vi "RecordDataToEventProgressCounterUp.vi"(10 "RecordData":string[][](array[string]), 11 "EventProgressDataInput":string[][](array[string])) -> (3 "EventProgressDataOutput":string[][](array[string]))   [LabVIEW 2017]
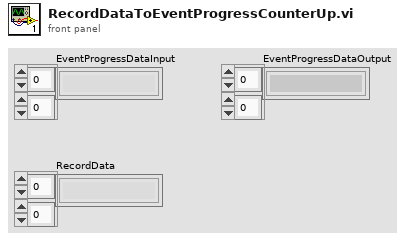
[diagram p1: front panel]
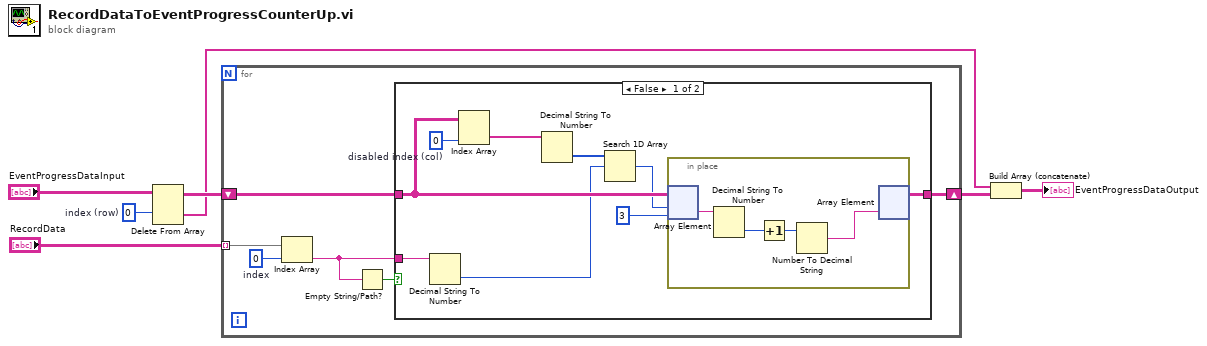
[diagram p0: block diagram]
diagram:
  w3 = 0  # index (row)
  n1 = Delete From Array "Delete From Array"(array="EventProgressDataInput", index (row)=w3) -> (deleted portion=w1:string[], array with subset deleted=w5:string[][])  [unwired: 2 in]
  n2 = for {
    tunnel: "RecordData" -> [w13] mode=indexing
    shift-right: [w10] -> w6
    shift-left: w5 -> [w12]
    w11 = 0  # index
    n3 = Index Array "Index Array"(array=w13, index=w11) -> (element=w9:string)
    n4 = Empty String/Path?(string/path=w9) -> (empty?=w8:bool)
    n5 = case shown="False" w8 {
      tunnel: w12 -> [w21 w27]
      tunnel: [w17 w27] -> w10
      tunnel: w9 -> [w14 _]
      frame False {
        w22 = 0  # disabled index (col)
        n6 = Decimal String To Number(string=w14) -> (number=w18:i32)  [unwired: 2 in, 1 out]
        n7 = Index Array "Index Array"(array=w21, index (col)=w22) -> (element=w20:string[])  [unwired: 1 in]
        n8 = Decimal String To Number(string=w20) -> (number=w19:i32[])  [unwired: 2 in, 1 out]
        n9 = Search 1D Array(1D array=w19, element=w18) -> (index of element=w16:i32)  [unwired: 1 in]
        n10 = in-place {
          n11 = in-place-array #1(w21, w16, 3) -> (w26:string)
          n12 = Decimal String To Number(string=w26) -> (number=w25:i32)  [unwired: 2 in, 1 out]
          n13 = Increment(x=w25) -> (x+1=w23:i32)
          n14 = Number To Decimal String(number=w23) -> (decimal integer string=w24:string)  [unwired: 1 in]
          n15 = in-place-array #1(w24) -> (w17:string[][])  [unwired: 2 out]
        }
      }
      frame True {
      }
    }
  }
  n16 = Build Array (concatenate) "Build Array"(w1, w6) -> (→"EventProgressDataOutput":string[][])
